vi "capex instrument control.vi"(0 "Keithley2268Lib.IKeithley2268":refnum<k7>, 4 "VISA resource name":refnum<visa-resource-name>, 6 "Bool in":bool[](array[boolean]), 7 "error in":errorcluster, 8 "Value in":dbl[](array[numeric]), 9 "Module":dbl=5.0, 10 "read/write":enum16{"read", "write"}(ring), 11 "Subsystem":T1(ring)=enum."temperature") -> (2 "Bool out":bool[](array[boolean]), 3 "Value out":dbl[](array[numeric]), 5 "error out":errorcluster)   [LabVIEW 2013]
uses:
  <vilib>/DAQmx/read.llb/DAQmx Read (Digital 1D Bool NChan 1Samp 1Line).vi
  <vilib>/DAQmx/write.llb/DAQmx Write (Digital 1D Bool NChan 1Samp 1Line).vi
  <vilib>/DAQmx/read.llb/DAQmx Read (Analog 2D DBL NChan NSamp).vi
  <vilib>/DAQmx/read.llb/DAQmx Read (Analog 1D DBL NChan 1Samp).vi
  <vilib>/DAQmx/write.llb/DAQmx Write (Analog 1D DBL NChan 1Samp).vi
  <vilib>/DAQmx/create/channels.llb/DAQmx Create Channel (DI-Digital Input).vi
  <vilib>/DAQmx/miscellaneous.llb/DAQmx Fill In Error Info.vi
  <vilib>/DAQmx/create/channels.llb/DAQmx Create Channel (DO-Digital Output).vi
  <vilib>/DAQmx/create/channels.llb/DAQmx Create Channel (AI-Temperature-Thermocouple).vi
  <vilib>/DAQmx/configure/timing.llb/DAQmx Timing (Sample Clock).vi
  <vilib>/DAQmx/create/channels.llb/DAQmx Create Channel (AI-Voltage-Basic).vi
  <vilib>/DAQmx/create/channels.llb/DAQmx Create Channel (AO-Voltage-Basic).vi
  <resource>/objmgr/daqmx.rc
  <instrlib>/APS-7000 Series/APS-7000 Series.lvlib
panel:
  in  "TC milliseconds to wait":u32=500
  out "Numeric 2":i32=12
  out "Numeric":i32=6
  in  "stop 5":bool
  in  "stop":bool
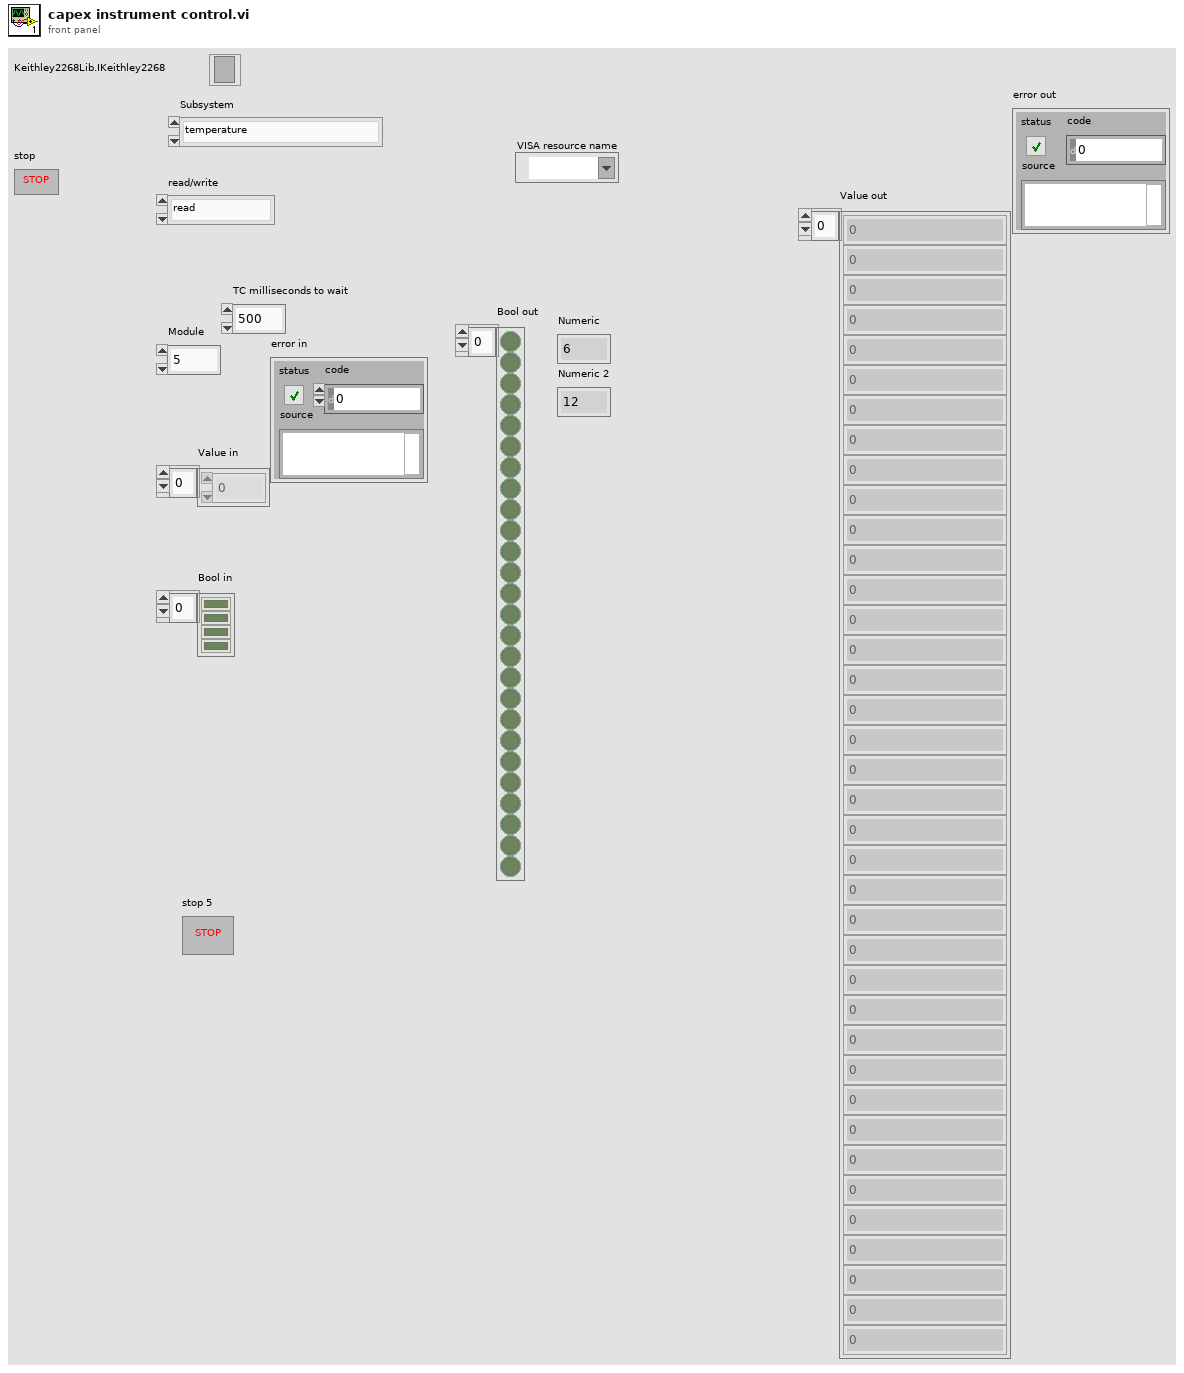
[diagram p1: front panel]
types:
  T1 = enum16{"Chiller", "Chamber", "DC power", "AC power", "GPIO", "temperature", "relays", "analog"}
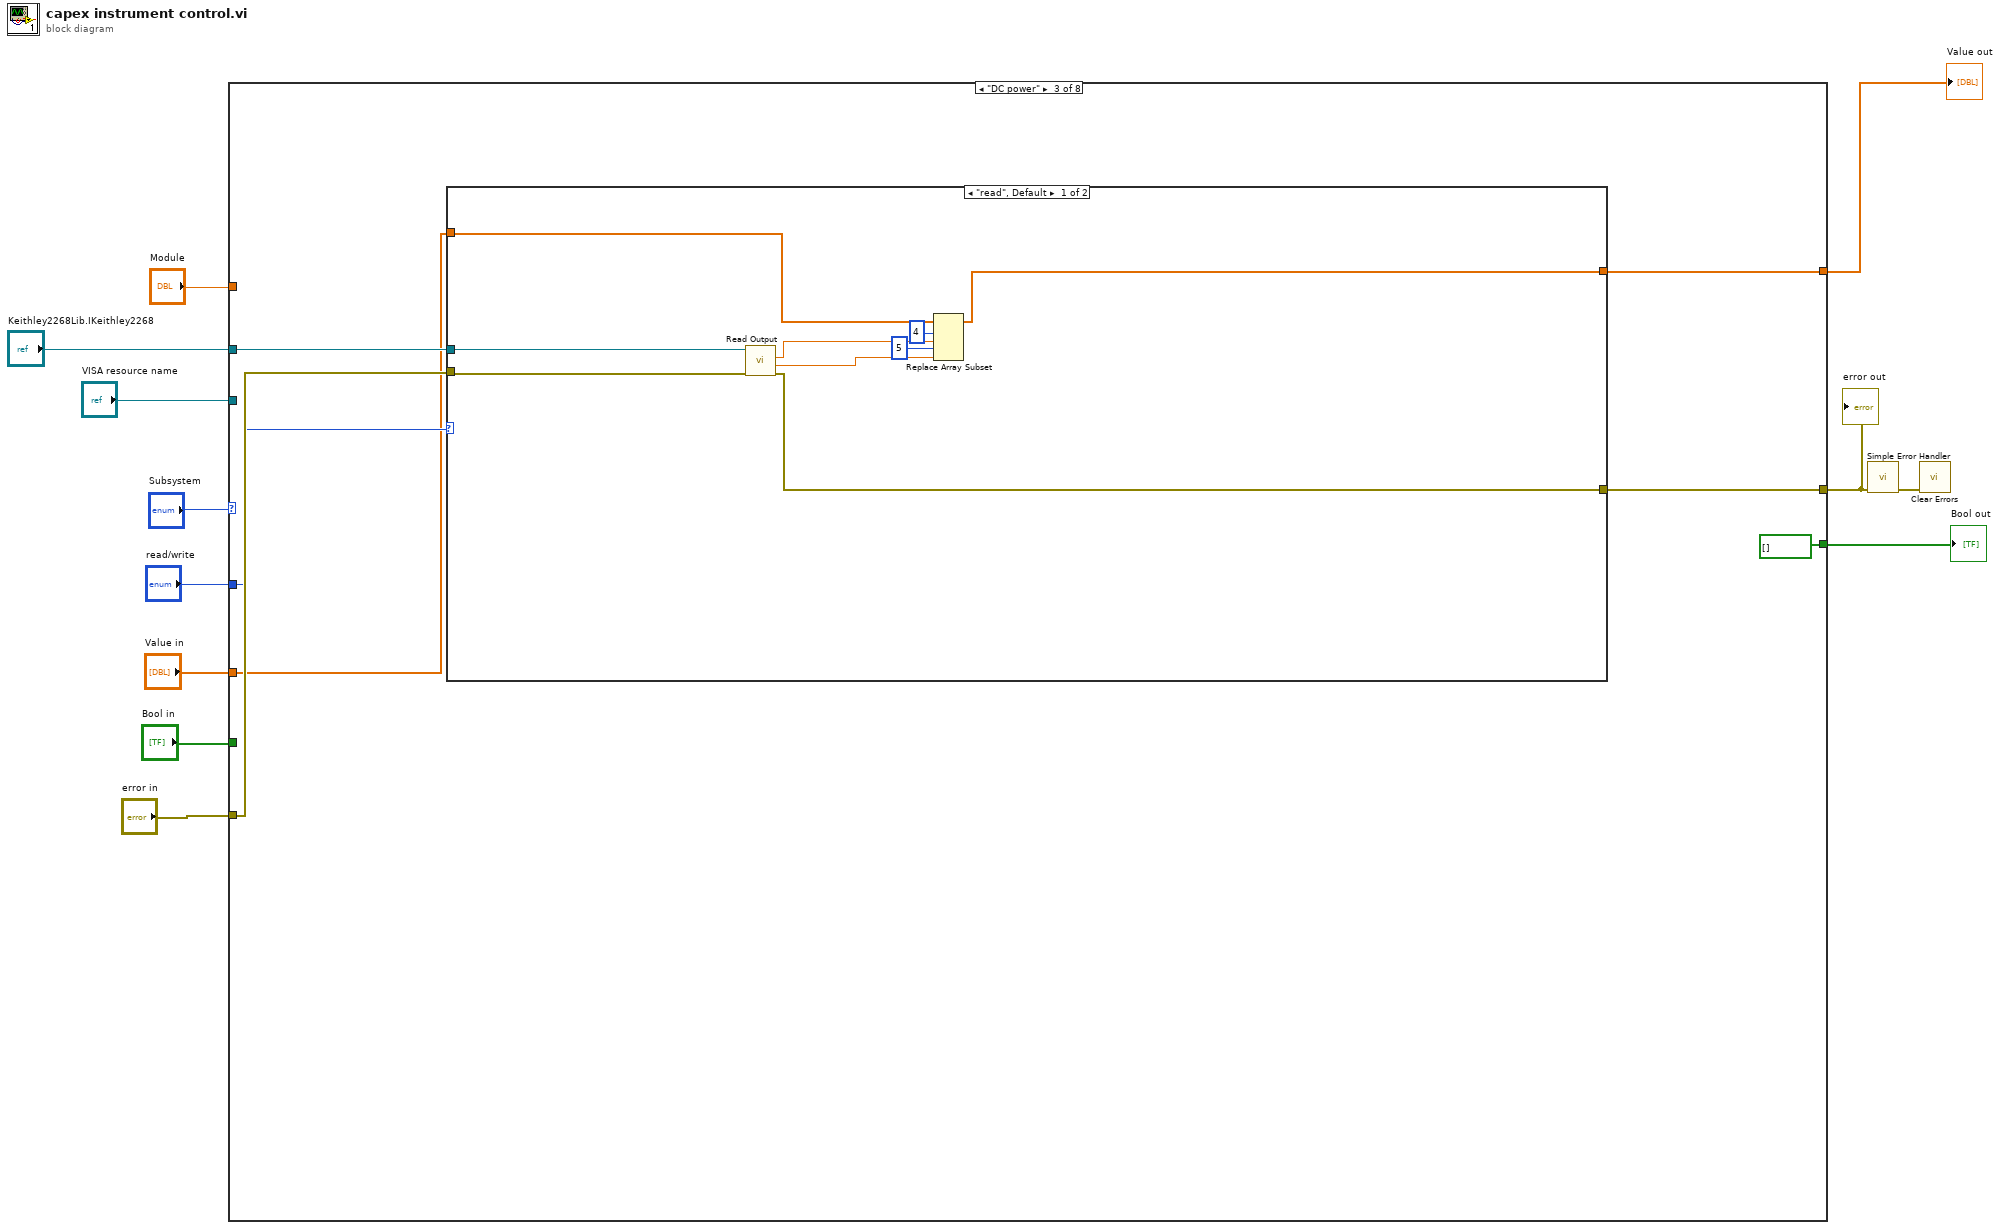
[diagram p0: block diagram]
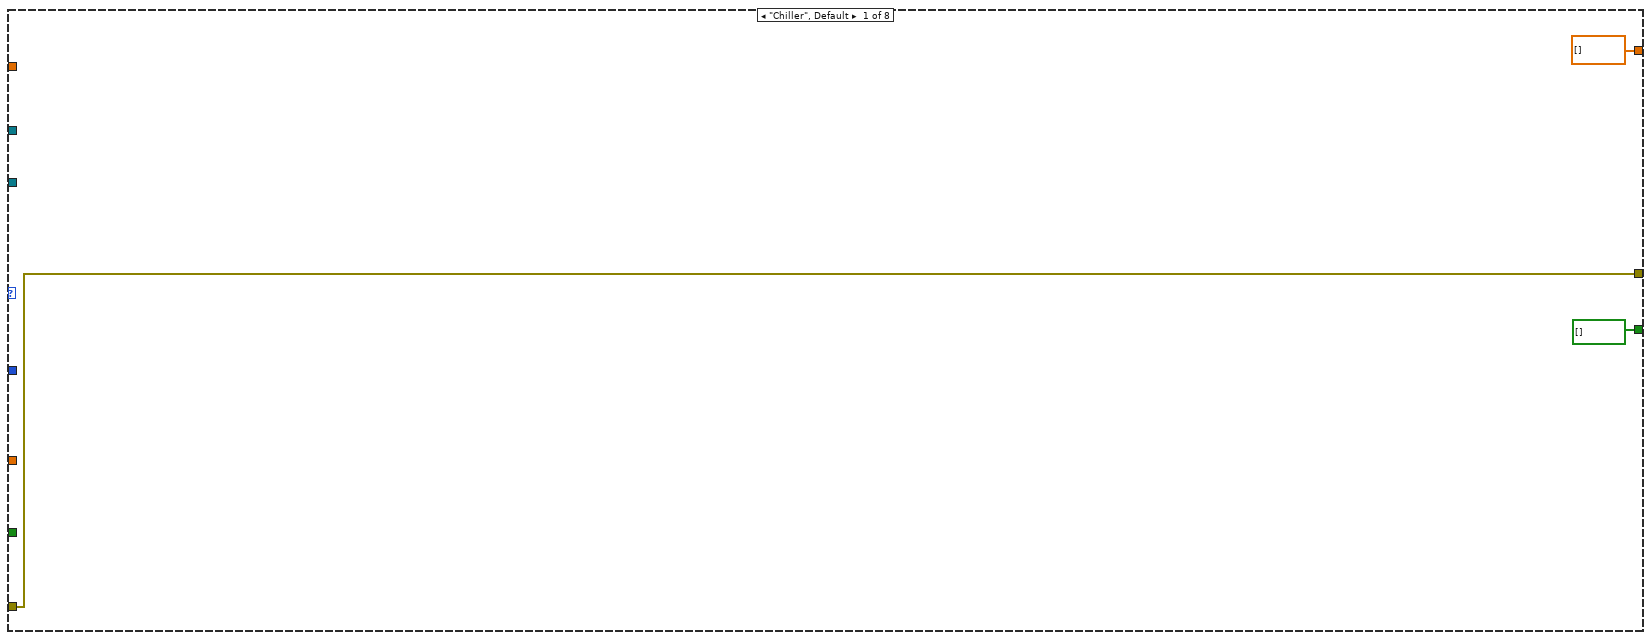
[diagram p2: hidden frame]
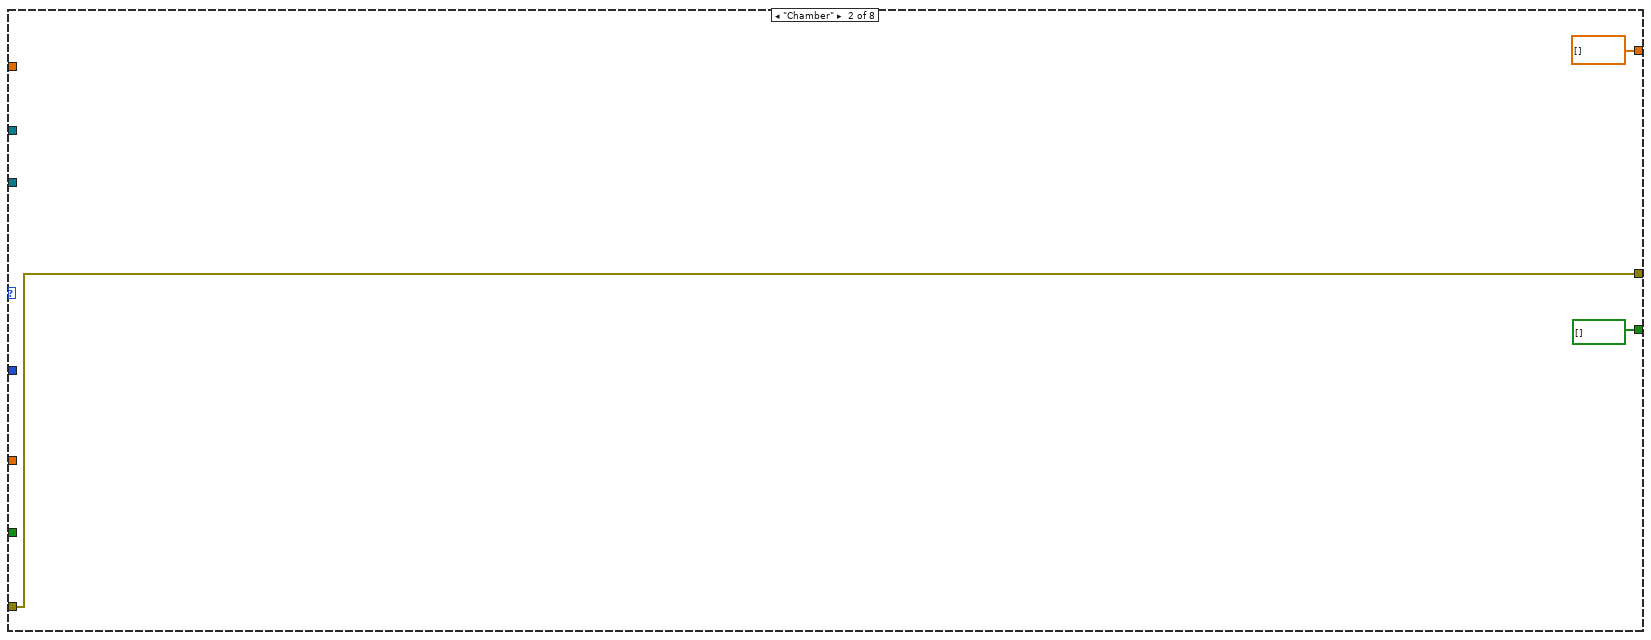
[diagram p3: hidden frame]
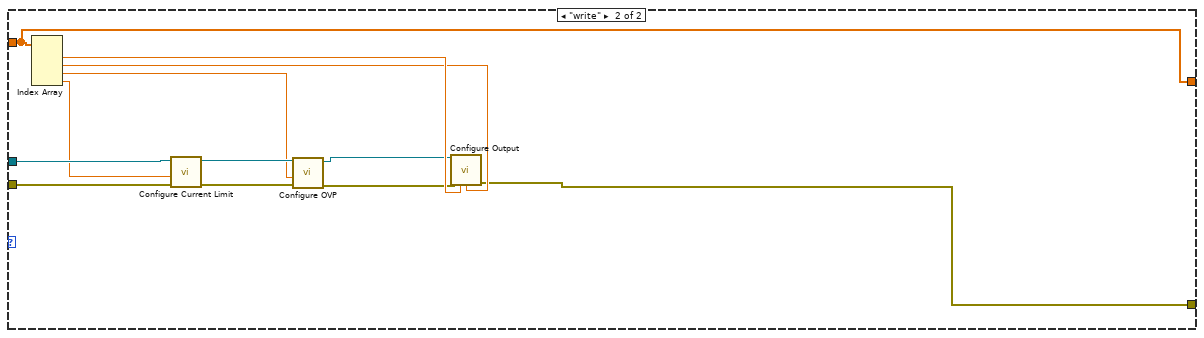
[diagram p4: hidden frame]
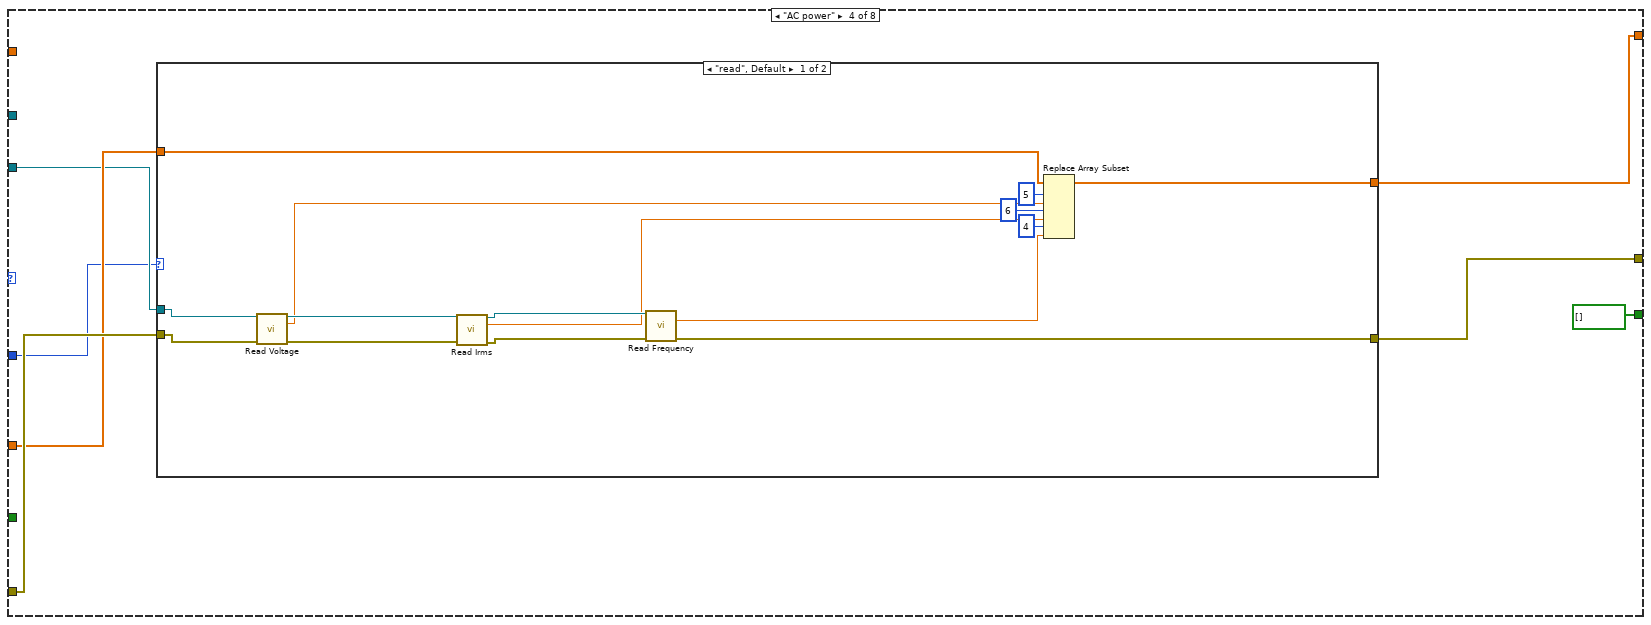
[diagram p5: hidden frame]
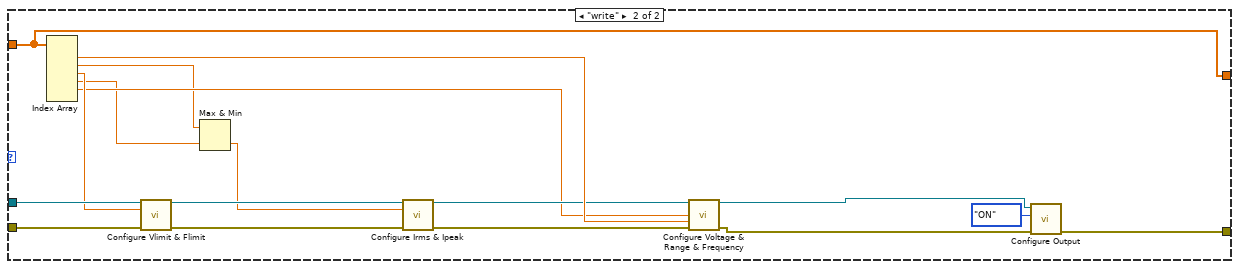
[diagram p6: hidden frame]
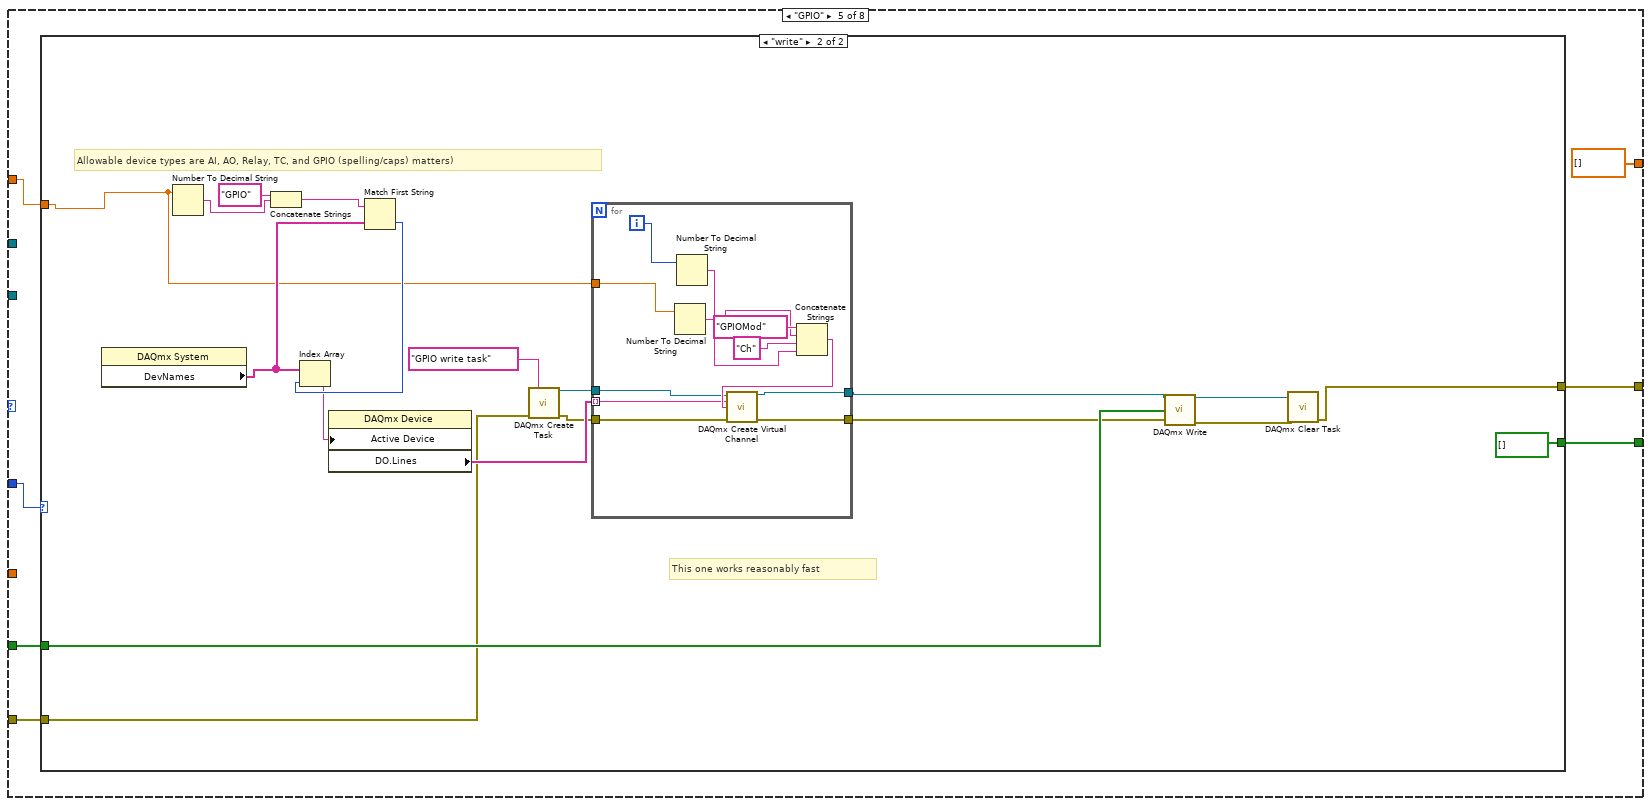
[diagram p7: hidden frame]
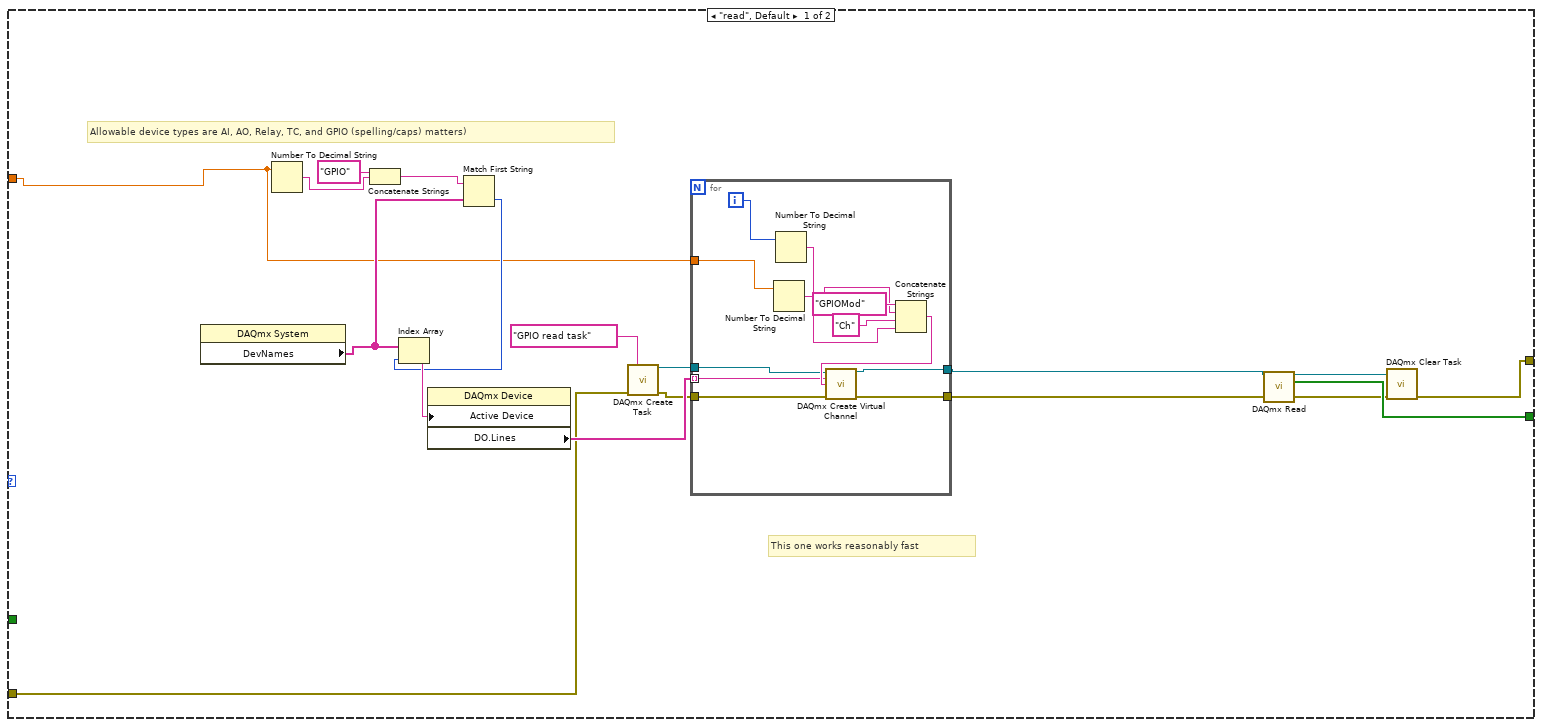
[diagram p8: hidden frame]
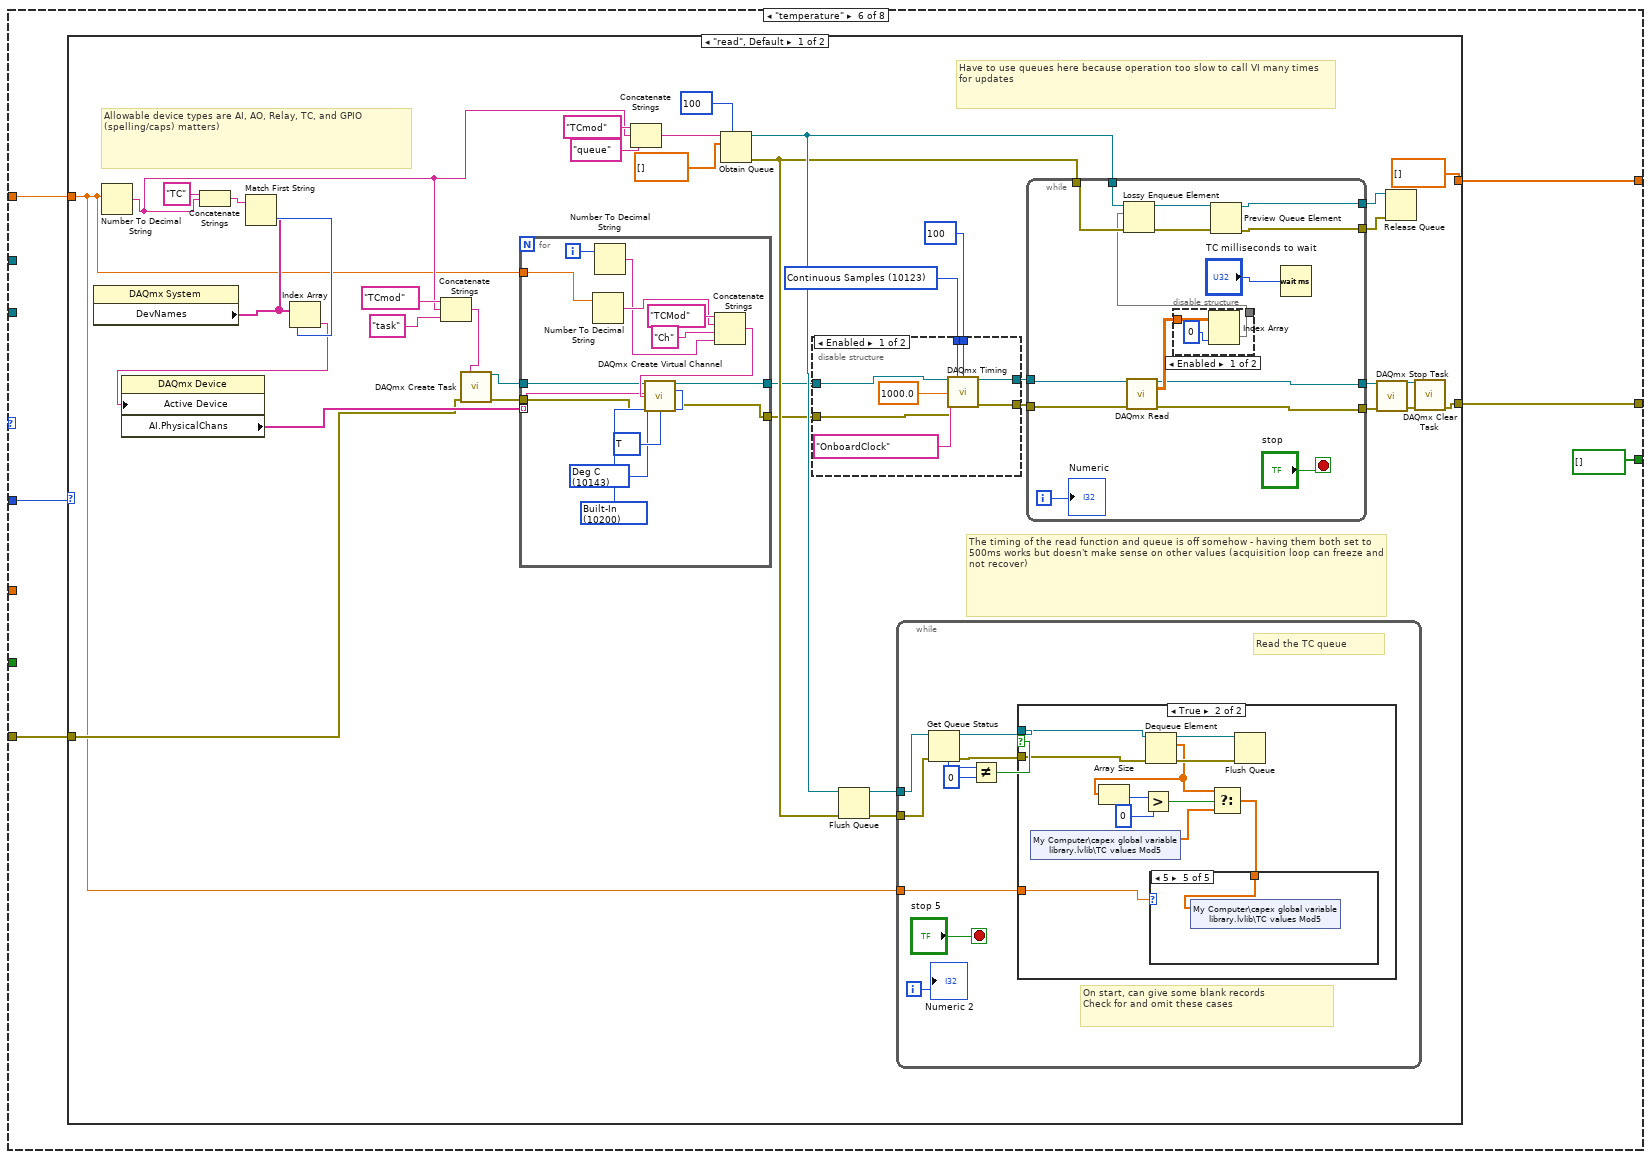
[diagram p9: hidden frame]
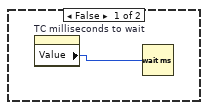
[diagram p11: hidden frame]
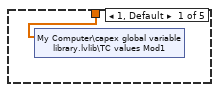
[diagram p12: hidden frame]
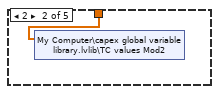
[diagram p13: hidden frame]
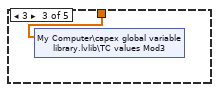
[diagram p14: hidden frame]
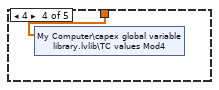
[diagram p15: hidden frame]
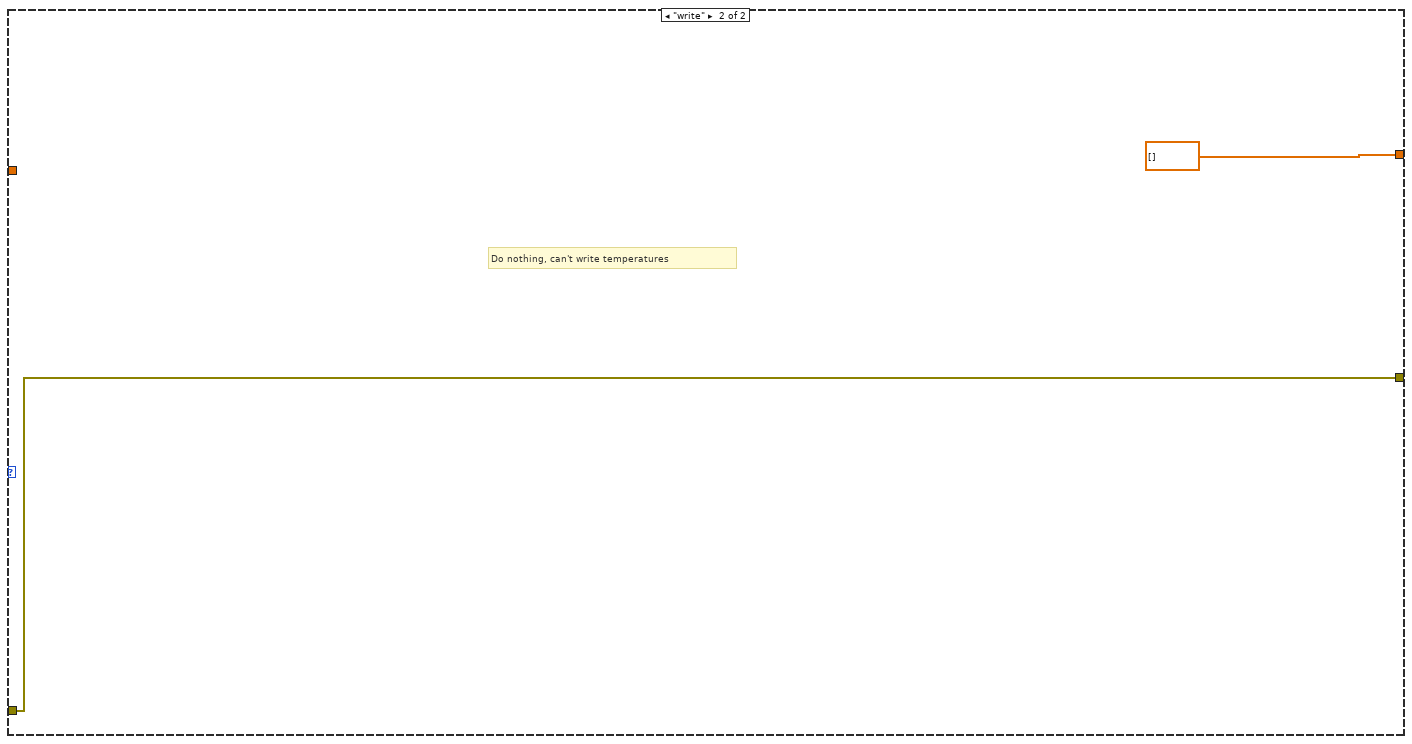
[diagram p17: hidden frame]
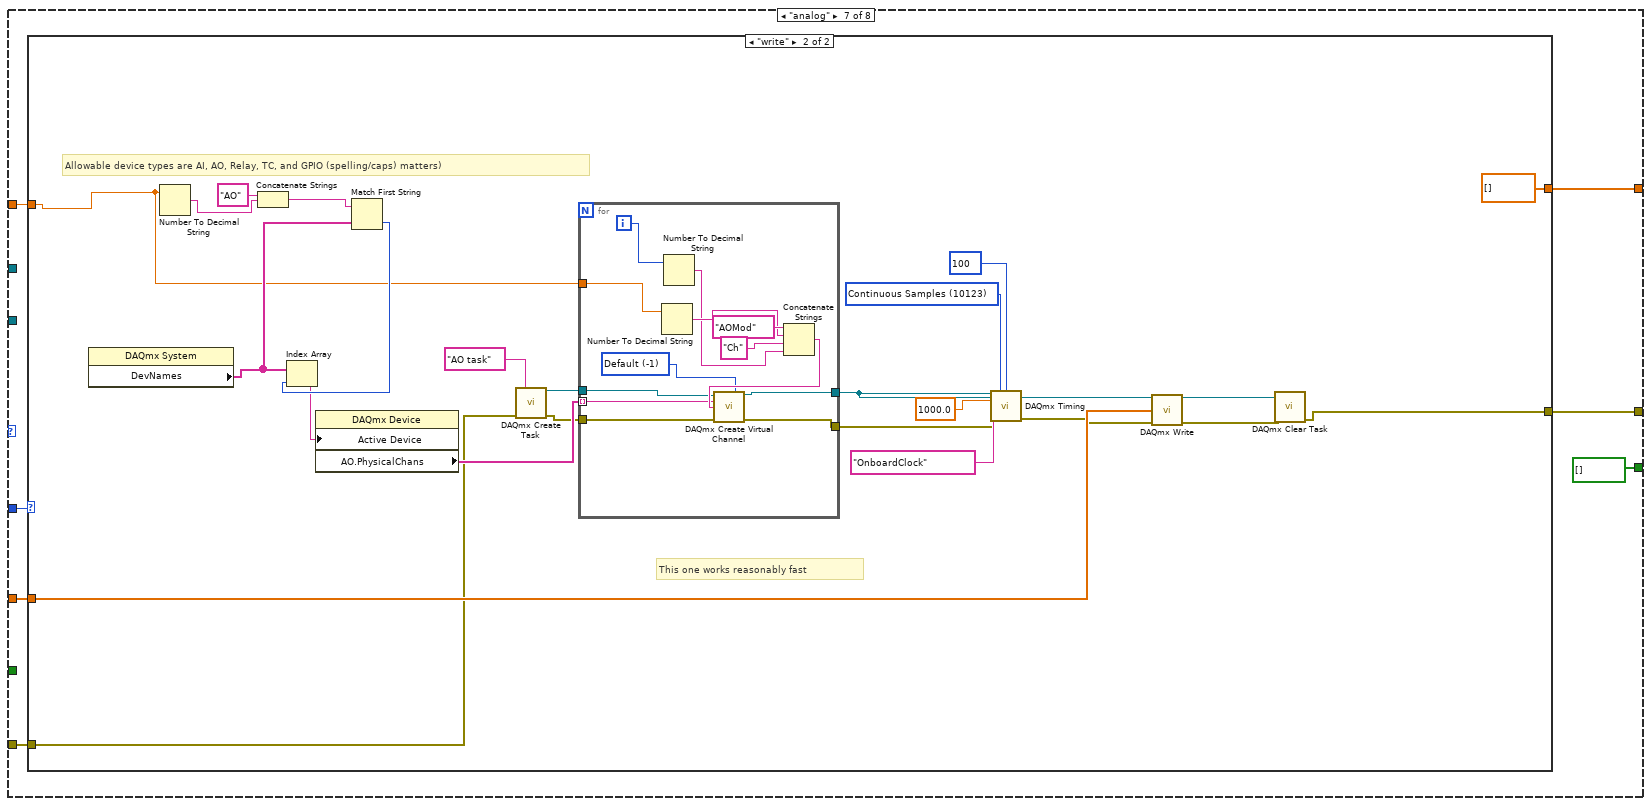
[diagram p18: hidden frame]
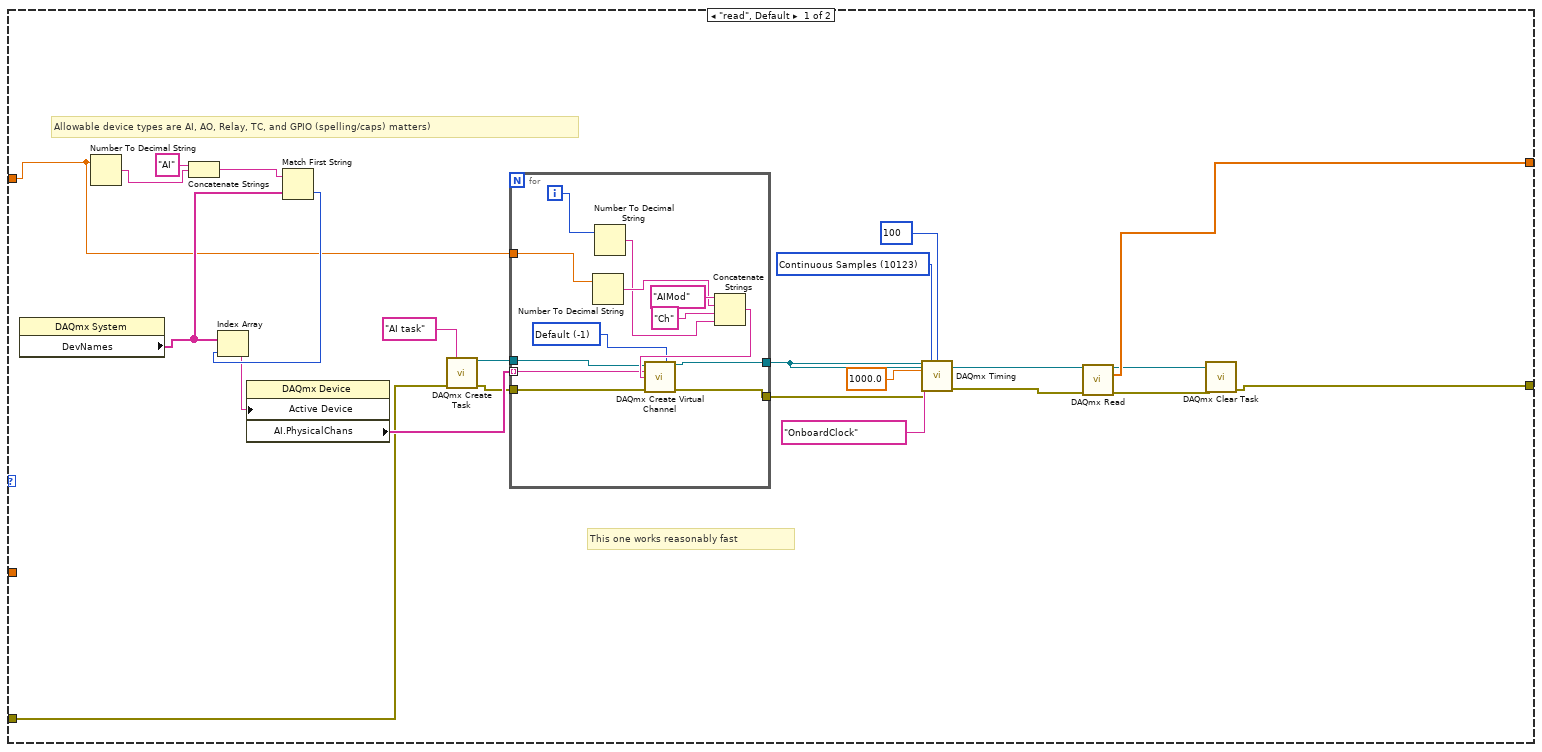
[diagram p19: hidden frame]
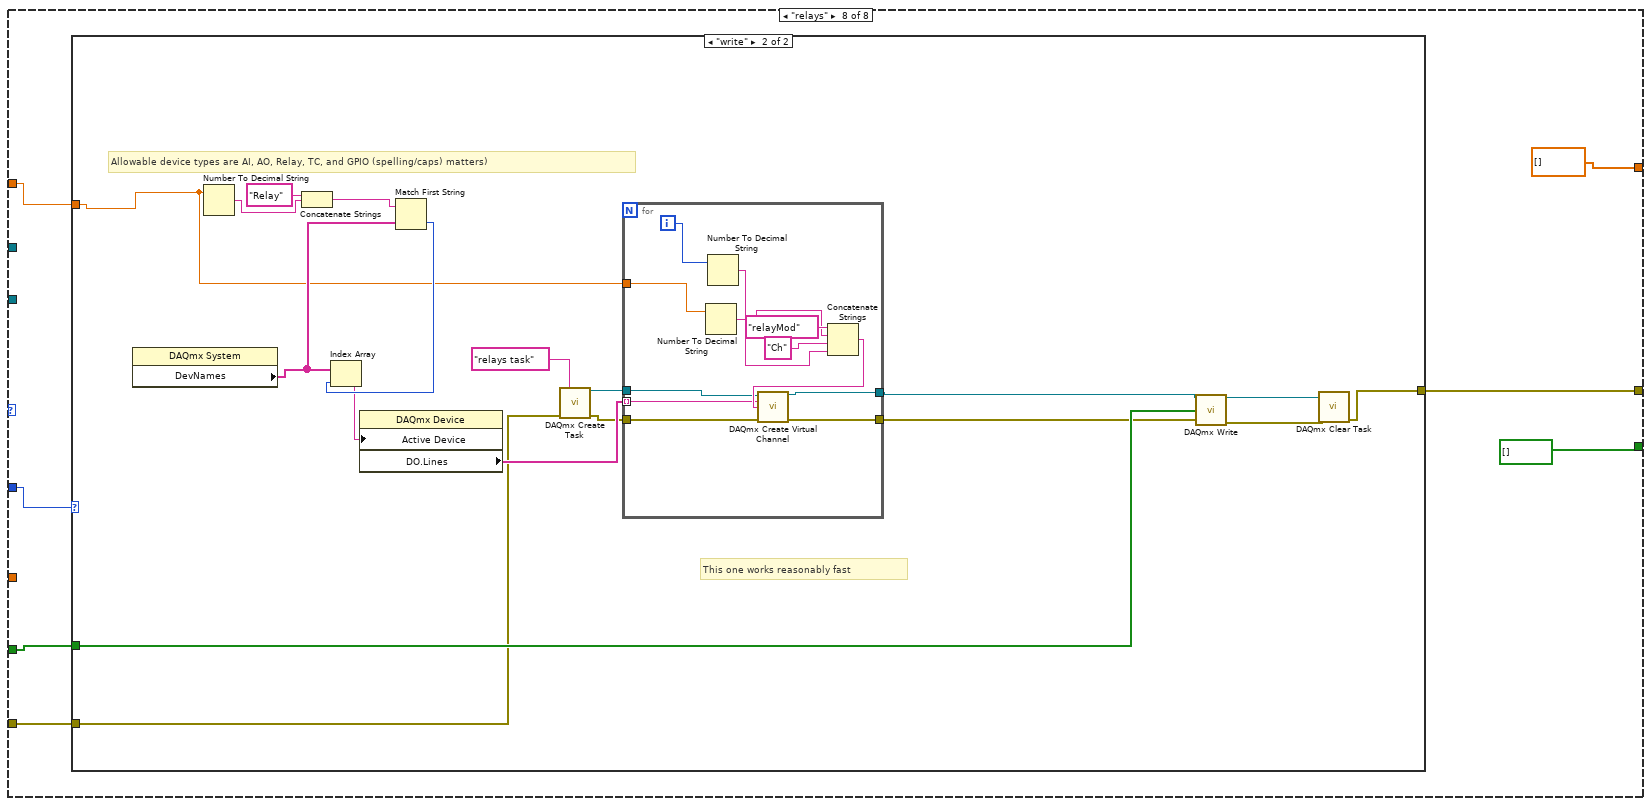
[diagram p20: hidden frame]
diagram:
  n1 = case shown="\"DC power\"" "Subsystem" {
    tunnel: "read/write" -> [_ _ w21 w48 w88 w159 w276 w352]
    tunnel: "Module" -> [_ _ _ _ w91 w158 w274 w356]
    tunnel: [dbl[] [] dbl[] [] w20 w47 dbl[] [] w157 w275 dbl[] []] -> w9
    tunnel: "Value in" -> [_ _ w19 w50 _ _ w273 _]
    tunnel: "Bool in" -> [_ _ _ _ w90 _ _ w355]
    tunnel: [bool[] [] ("data") bool[] [] ("data") bool[] [] ("data") bool[] [] ("data") w89 bool[] [] ("data") bool[] [] ("data") bool[] [] ("data")] -> w6
    tunnel: "error in" -> [w13 w16 w23 w52 w87 w155 w271 w351]
    tunnel: [w13 w16 w22 w51 w86 w154 w270 w350] -> w4
    tunnel: "VISA resource name" -> [_ _ _ w49 _ _ _ _]
    tunnel: "Keithley2268Lib.IKeithley2268" -> [_ _ w24 _ _ _ _ _]
    frame "Chiller", Default {
    }
    frame "Chamber" {
    }
    frame "DC power" {
      n2 = case shown="\"read\", Default" w21 {
        tunnel: w19 -> [w32 w35]
        tunnel: w24 -> [w34 w46]
        tunnel: w23 -> [w33 w39]
        tunnel: [w26 w36] -> w22
        tunnel: [w27 w35] -> w20
        frame "read", Default {
          n3 = call <instrlib>:"Read Output.vi"("error in (no error)"=w33, "Keithley2268Lib.IKeithley2268"=w34) -> ("error out"=w26:errorcluster, "Current Level (A)"=w29:dbl, "Voltage Level (V)"=w31:dbl)  [unwired: 6 in, 1 out]
          n4 = Replace Array Subset(array=w32, new element #1=w31, index #1=4 ("index"), new element #2=w29, index #2=5 ("index")) -> (w27:dbl[])
        }
        frame "write" {
          n5 = Index Array(array=w35) -> (element #1=w45:dbl, element #2=w44:dbl, element #3=w40:dbl, element #4=w41:dbl)  [unwired: 4 in]
          n6 = call <instrlib>:"Configure Current Limit.vi"("error in (no error)"=w39, "Current Limit (V)"=w41, "Keithley2268Lib.IKeithley2268"=w46) -> ("error out"=w38:errorcluster, "Keithley2268Lib.IKeithley2268"=w43:refnum<k7>)  [unwired: 7 in]
          n7 = call <instrlib>:"Configure OVP.vi"("error in (no error)"=w38, "OVP Level (V)"=w40, "Keithley2268Lib.IKeithley2268"=w43) -> ("error out"=w37:errorcluster, "Keithley2268Lib.IKeithley2268"=w42:refnum<k7>)  [unwired: 7 in]
          n8 = call <instrlib>:"Configure Output.vi"("Keithley2268Lib.IKeithley2268"=w42, "error in (no error)"=w37, "Voltage Level (V)"=w45, "Current Level (A)"=w44) -> ("error out"=w36:errorcluster)  [unwired: 10 in, 1 out]
        }
      }
    }
    frame "AC power" {
      n9 = case shown="\"read\", Default" w48 {
        tunnel: w52 -> [w64 w85]
        tunnel: [w61 w81] -> w51
        tunnel: w50 -> [w68 w69]
        tunnel: w49 -> [w67 w78]
        tunnel: [w54 w69] -> w47
        frame "read", Default {
          n10 = call <instrlib>:"Read Voltage.vi"("VISA session"=w67, "error in"=w64) -> ("dup VISA session"=w66:refnum<visa-resource-name>, "ACV?"=w60:dbl, "error out"=w63:errorcluster)  [unwired: 9 in, 2 out]
          n11 = call <instrlib>:"Read Irms.vi"("VISA in"=w66, "error in"=w63) -> ("VISA out"=w65:refnum<visa-resource-name>, "Irms? (Arms)"=w59:dbl, "error out"=w62:errorcluster)  [unwired: 9 in, 2 out]
          n12 = call <instrlib>:"Read Frequency.vi"("VISA session"=w65, "error in"=w62) -> ("Freq? (Hz)"=w58:dbl, "error out"=w61:errorcluster)  [unwired: 9 in, 3 out]
          n13 = Replace Array Subset(array=w68, new element #1=w60, index #1=5 ("index"), new element #2=w59, index #2=6 ("index"), new element #3=w58, index #3=4 ("index")) -> (w54:dbl[])
        }
        frame "write" {
          n14 = Index Array(array=w69) -> (element #1=w79:dbl, element #2=w72:dbl, element #3=w74:dbl, element #4=w71:dbl, element #5=w73:dbl)  [unwired: 6 in, 1 out]
          n15 = call <instrlib>:"Configure Vlimit & Flimit.vi"("VISA in"=w78, "Vlimit (Vrms)"=w74, "error in"=w85) -> ("VISA out"=w77:refnum<visa-resource-name>, "error out"=w84:errorcluster)  [unwired: 5 in, 6 out]
          n16 = Max & Min(x=w72, y=w71) -> (min(x,y)=w70:dbl)  [unwired: 1 out]
          n17 = call <instrlib>:"Configure Irms & Ipeak.vi"("VISA in"=w77, "Irms (A)"=w70, "error in"=w84) -> ("VISA out"=w76:refnum<visa-resource-name>, "error out"=w83:errorcluster)  [unwired: 5 in, 6 out]
          n18 = call <instrlib>:"Configure Voltage & Range & Frequency.vi"("VISA in"=w76, "FREQ"=w73, "ACV"=w79, "error in"=w83) -> ("VISA out"=w75:refnum<visa-resource-name>, "error out"=w82:errorcluster)  [unwired: 3 in, 7 out]
          n19 = call <instrlib>:"Configure Output.vi"("error in"=w82, "Output ON/OFF"=enum16{"OFF", "ON"}."ON", "VISA in"=w75) -> ("error out"=w81:errorcluster)  [unwired: 6 in, 2 out]
        }
      }
    }
    frame "GPIO" {
      n20 = case shown="\"write\"" w88 {
        tunnel: w91 -> [w100 w131]
        tunnel: w90 -> [_ w130]
        tunnel: [w99 bool[] [] ("data")] -> w89
        tunnel: w87 -> [w97 w127]
        tunnel: [w93 w123] -> w86
        frame "read", Default {
          # "Allowable device types are AI, AO, Relay, TC, and GPIO (spelling/caps) matters)"
          # "This one works reasonably fast"
          n21 = property class="DAQmx System"() -> ("DevNames"=w105:tag[])  [unwired: 2 in, 2 out]
          n22 = Number To Decimal String(number=w100) -> (decimal integer string=w102:string)  [unwired: 1 in]
          n23 = Concatenate Strings("GPIO" ("string"), w102) -> (w103:string)
          n24 = Match First String(2:w105, 3:w103) -> (0:w104:i32)  [unwired: 1 out]
          n25 = Index Array(array=w105, index=w104) -> (element=w106:tag)
          n26 = property class="DAQmx Device"("Active Device"=w106) -> ("DO.Lines"=w109:tag[])  [unwired: 2 in, 2 out]
          n27 = call <vilib>:"DAQmx Create Task.vi"("new task name"="GPIO read task", "error in"=w97) -> ("task out"=w107:refnum<k21>, "error out"=w96:errorcluster)  [unwired: 12 in]
          n28 = for {
            tunnel: w100 -> [w117]
            tunnel: w107 -> [w116]
            tunnel: [w115] -> w98
            tunnel: w109 -> [w114] mode=indexing
            tunnel: w96 -> [w112]
            tunnel: [w111] -> w95
            i -> [w113]
            n29 = Number To Decimal String(number=w117) -> (decimal integer string=w121:string)  [unwired: 1 in]
            n30 = Number To Decimal String(number=w113) -> (decimal integer string=w120:string)  [unwired: 1 in]
            n31 = Concatenate Strings("GPIOMod" ("string"), w121, "Ch" ("string"), w120) -> (w118:string)
            n32 = call-poly <vilib>:"DAQmx Create Virtual Channel.vi"("task in"=w116, "lines"=w114, "name to assign"=w118, "error in"=w112) -> ("task out"=w115:refnum<k21>, "error out"=w111:errorcluster)  [unwired: 10 in]
          }
          n33 = call-poly <vilib>:"DAQmx Read.vi"("task/channels in"=w98, "error in"=w95) -> ("task out"=w108:refnum<k21>, "data"=w99:bool[], "error out"=w94:errorcluster)  [unwired: 11 in]
          n34 = call <vilib>:"DAQmx Clear Task.vi"("task in"=w108, "error in"=w94) -> ("error out"=w93:errorcluster)  [unwired: 13 in]
        }
        frame "write" {
          # "Allowable device types are AI, AO, Relay, TC, and GPIO (spelling/caps) matters)"
          # "This one works reasonably fast"
          n35 = property class="DAQmx System"() -> ("DevNames"=w137:tag[])  [unwired: 2 in, 2 out]
          n36 = Number To Decimal String(number=w131) -> (decimal integer string=w140:string)  [unwired: 1 in]
          n37 = Concatenate Strings("GPIO" ("string"), w140) -> (w139:string)
          n38 = Match First String(2:w137, 3:w139) -> (0:w138:i32)  [unwired: 1 out]
          n39 = Index Array(array=w137, index=w138) -> (element=w136:tag)
          n40 = property class="DAQmx Device"("Active Device"=w136) -> ("DO.Lines"=w133:tag[])  [unwired: 2 in, 2 out]
          n41 = call <vilib>:"DAQmx Create Task.vi"("new task name"="GPIO write task", "error in"=w127) -> ("task out"=w135:refnum<k21>, "error out"=w126:errorcluster)  [unwired: 12 in]
          n42 = for {
            tunnel: w131 -> [w148]
            tunnel: w135 -> [w147]
            tunnel: [w146] -> w128
            tunnel: w133 -> [w145] mode=indexing
            tunnel: w126 -> [w143]
            tunnel: [w142] -> w125
            i -> [w144]
            n43 = Number To Decimal String(number=w148) -> (decimal integer string=w152:string)  [unwired: 1 in]
            n44 = Number To Decimal String(number=w144) -> (decimal integer string=w151:string)  [unwired: 1 in]
            n45 = Concatenate Strings("GPIOMod" ("string"), w152, "Ch" ("string"), w151) -> (w149:string)
            n46 = call-poly <vilib>:"DAQmx Create Virtual Channel.vi"("task in"=w147, "lines"=w145, "name to assign"=w149, "error in"=w143) -> ("task out"=w146:refnum<k21>, "error out"=w142:errorcluster)  [unwired: 10 in]
          }
          n47 = call-poly <vilib>:"DAQmx Write.vi"("task/channels in"=w128, "data"=w130, "error in"=w125) -> ("task out"=w134:refnum<k21>, "error out"=w124:errorcluster)  [unwired: 10 in, 1 out]
          n48 = call <vilib>:"DAQmx Clear Task.vi"("task in"=w134, "error in"=w124) -> ("error out"=w123:errorcluster)  [unwired: 13 in]
        }
      }
    }
    frame "temperature" {
      n49 = case shown="\"read\", Default" w159 {
        tunnel: w158 -> [w174 _]
        tunnel: [dbl[] [] dbl[] []] -> w157
        tunnel: w155 -> [w190 w268]
        tunnel: [w169 w268] -> w154
        frame "read", Default {
          w168 = 10123 items=["Finite Samples"=10178, "Continuous Samples"=10123, "Hardware Timed Single Point"=12522] ("sample mode")
          # "The timing of the read function and queue is off somehow - having them both set to 500ms works but doesn't make sense on other values (acquisition loop can freeze and not recover)"
          # "Have to use queues here because operation too slow to call VI many times for updates"
          # "Allowable device types are AI, AO, Relay, TC, and GPIO (spelling/caps) matters)"
          n50 = property class="DAQmx System"() -> ("DevNames"=w194:tag[])  [unwired: 2 in, 2 out]
          n51 = Number To Decimal String(number=w174) -> (decimal integer string=w181:string)  [unwired: 1 in]
          n52 = Concatenate Strings("TC" ("string"), w181) -> (w178:string)
          n53 = Match First String(2:w194, 3:w178) -> (0:w195:i32)  [unwired: 1 out]
          n54 = Index Array(array=w194, index=w195) -> (element=w193:tag)
          n55 = property class="DAQmx Device"("Active Device"=w193) -> ("AI.PhysicalChans"=w191:tag[])  [unwired: 2 in, 2 out]
          n56 = Concatenate Strings("TCmod" ("new task name"), w181, "task" ("string")) -> (w179:string)
          n57 = call <vilib>:"DAQmx Create Task.vi"("new task name"=w179, "error in"=w190) -> ("task out"=w192:refnum<k21>, "error out"=w189:errorcluster)  [unwired: 12 in]
          n58 = for {
            tunnel: w174 -> [w267]
            tunnel: [w258] -> w165
            tunnel: w192 -> [w256]
            tunnel: w191 -> [w255] mode=indexing
            tunnel: w189 -> [w254]
            tunnel: [w253] -> w166
            i -> [w257]
            w259 = 10200 items=["Built-In"=10200, "Constant Value"=10116, "Channel"=10113] ("cjc source")
            w260 = 10143 items=["Deg C"=10143, "Deg F"=10144, "Kelvins"=10325, "Deg R"=10145, "From Custom Scale"=10065] ("units")
            w266 = 10086 items=["J"=10072, "K"=10073, "N"=10077, "R"=10082, "S"=10085, "T"=10086, "B"=10047, "E"=10055] ("thermocouple type")
            n59 = Number To Decimal String(number=w267) -> (decimal integer string=w264:string)  [unwired: 1 in]
            n60 = Number To Decimal String(number=w257) -> (decimal integer string=w263:string)  [unwired: 1 in]
            n61 = Concatenate Strings("TCMod" ("string"), w264, "Ch" ("string"), w263) -> (w261:string)
            n62 = call-poly <vilib>:"DAQmx Create Virtual Channel.vi"("task in"=w256, "physical channels"=w255, "cjc source"=w259, "name to assign"=w261, "units"=w260, "error in"=w254, "thermocouple type"=w266) -> ("task out"=w258:refnum<k21>, "error out"=w253:errorcluster)  [unwired: 7 in]
          }
          n63 = Concatenate Strings("TCmod" ("string"), w181, "queue" ("string")) -> (w186:string)
          n64 = Obtain Queue(max queue size (-1, unlimited)=100, name (unnamed)=w186, element data type=dbl[] [] ("Value out 2")) -> (queue out=w176:refnum<queue>, error out=w175:errorcluster)  [unwired: 2 in, 1 out]
          n65 = disable-structure shown="Enabled" {
            disable-tunnel: w168 -> [w202 _]
            disable-tunnel: 100 ("samples per channel") -> [w201 _]
            disable-tunnel: w166 -> [w200 w205]
            disable-tunnel: w165 -> [w199 w206]
            disable-tunnel: [w198 w206] -> w164
            disable-tunnel: [w197 w205] -> w163
            frame Enabled {
              n66 = call-poly <vilib>:"DAQmx Timing.vi"("task/channels in"=w199, "sample mode"=w202, "samples per channel"=w201, "rate"=1000.0, "source"=tag "OnboardClock", "error in"=w200) -> ("task out"=w198:refnum<k21>, "error out"=w197:errorcluster)  [unwired: 8 in]
            }
            frame Disabled {
            }
          }
          n67 = Flush Queue(queue=w176, error in (no error)=w175) -> (queue out=w161:refnum<queue>, error out=w160:errorcluster)  [unwired: 1 out]
          n68 = while {
            tunnel: w161 -> [w213]
            tunnel: w160 -> [w212]
            tunnel: w174 -> [w208]
            i -> [w215]
            stop <- "stop 5" stop-if-true
            # "On start, can give some blank records\nCheck for and omit these cases"
            # "Read the TC queue"
            n69 = Get Queue Status(queue=w213, error in (no error)=w212) -> (queue out=w210:refnum<queue>, error out=w209:errorcluster, # elements in queue=w207:i32)  [unwired: 1 in, 5 out]
            n70 = Not Equal?(x=w207, y=0) -> (x != y?=w211:bool)
            n71 = case shown="True" w211 {
              tunnel: w210 -> [_ w226]
              tunnel: w209 -> [_ w225]
              tunnel: w208 -> [_ w224]
              frame False {
                n72 = property on="TC milliseconds to wait" class="DigNum (strict)"() -> ("Value"=w217:u32)  [unwired: 2 in, 2 out]
                n73 = Wait (ms)(milliseconds to wait=w217) -> ()  [unwired: 1 out]
              }
              frame True {
                n74 = shared-variable "My Computer\\capex global variable library.lvlib\\TC values Mod5"() -> (w218:dbl[])  [unwired: 1 in, 1 out]
                n75 = Dequeue Element(queue=w226, error in (no error)=w225) -> (queue out=w228:refnum<queue>, element=w220:dbl[], error out=w227:errorcluster)  [unwired: 1 in, 1 out]
                n76 = Array Size(array=w220) -> (size(s)=w223:i32)
                n77 = Greater?(x=w223, y=0) -> (0:w221:bool)
                n78 = Select(t=w220, s=w221, f=w218) -> (s? t:f=w219:dbl[])
                n79 = case shown="5" w224 {
                  tunnel: w219 -> [w229 w230 w231 w232 w233]
                  frame 1, Default {
                    n80 = shared-variable "My Computer\\capex global variable library.lvlib\\TC values Mod1"(w229) -> ()  [unwired: 1 in, 1 out]
                  }
                  frame 2 {
                    n81 = shared-variable "My Computer\\capex global variable library.lvlib\\TC values Mod2"(w230) -> ()  [unwired: 1 in, 1 out]
                  }
                  frame 3 {
                    n82 = shared-variable "My Computer\\capex global variable library.lvlib\\TC values Mod3"(w231) -> ()  [unwired: 1 in, 1 out]
                  }
                  frame 4 {
                    n83 = shared-variable "My Computer\\capex global variable library.lvlib\\TC values Mod4"(w232) -> ()  [unwired: 1 in, 1 out]
                  }
                  frame 5 {
                    n84 = shared-variable "My Computer\\capex global variable library.lvlib\\TC values Mod5"(w233) -> ()  [unwired: 1 in, 1 out]
                  }
                }
                n85 = Flush Queue(queue=w228, error in (no error)=w227) -> ()  [unwired: 3 out]
              }
            }
            "Numeric 2" <- w215
          }
          n86 = while {
            tunnel: [w236] -> w173
            tunnel: w163 -> [w240]
            tunnel: [w235] -> w172
            tunnel: w176 -> [w247]
            tunnel: [w245] -> w184
            tunnel: w175 -> [w246]
            tunnel: [w244] -> w183
            tunnel: w164 -> [w239]
            i -> [w241]
            stop <- "stop" stop-if-true
            n87 = call-poly <vilib>:"DAQmx Read.vi"("task/channels in"=w239, "error in"=w240) -> ("task out"=w236:refnum<k21>, "data"=w237:dbl[][], "error out"=w235:errorcluster)  [unwired: 11 in]
            n88 = disable-structure shown="Enabled" {
              disable-tunnel: [w251 w252] -> w238
              disable-tunnel: w237 -> [w249 w252]
              frame Enabled {
                n89 = Index Array(array=w249, index (col)=0 ("index (row)")) -> (element=w251:dbl[])  [unwired: 1 in]
              }
              frame Disabled {
              }
            }
            n90 = Lossy Enqueue Element(queue=w247, element=w238, error in (no error)=w246) -> (queue out=w243:refnum<queue>, error out=w242:errorcluster)  [unwired: 2 out]
            n91 = Preview Queue Element(queue=w243, error in (no error)=w242) -> (queue out=w245:refnum<queue>, error out=w244:errorcluster)  [unwired: 1 in, 2 out]
            n92 = Wait (ms)(milliseconds to wait="TC milliseconds to wait") -> ()  [unwired: 1 out]
            "Numeric" <- w241
          }
          n93 = call <vilib>:"DAQmx Stop Task.vi"("task/channels in"=w173, "error in"=w172) -> ("task out"=w171:refnum<k21>, "error out"=w170:errorcluster)  [unwired: 12 in]
          n94 = Release Queue(queue=w184, error in (no error)=w183) -> ()  [unwired: 1 in, 3 out]
          n95 = call <vilib>:"DAQmx Clear Task.vi"("task in"=w171, "error in"=w170) -> ("error out"=w169:errorcluster)  [unwired: 13 in]
        }
        frame "write" {
          # "Do nothing, can't write temperatures"
        }
      }
    }
    frame "analog" {
      n96 = case shown="\"write\"" w276 {
        tunnel: [w293 dbl[] []] -> w275
        tunnel: w274 -> [w292 w320]
        tunnel: w273 -> [_ w319]
        tunnel: w271 -> [w282 w318]
        tunnel: [w277 w313] -> w270
        frame "read", Default {
          w289 = 10123 items=["Finite Samples"=10178, "Continuous Samples"=10123, "Hardware Timed Single Point"=12522] ("sample mode")
          # "Allowable device types are AI, AO, Relay, TC, and GPIO (spelling/caps) matters)"
          # "This one works reasonably fast"
          n97 = property class="DAQmx System"() -> ("DevNames"=w295:tag[])  [unwired: 2 in, 2 out]
          n98 = Number To Decimal String(number=w292) -> (decimal integer string=w298:string)  [unwired: 1 in]
          n99 = Concatenate Strings("AI" ("string"), w298) -> (w297:string)
          n100 = Match First String(2:w295, 3:w297) -> (0:w296:i32)  [unwired: 1 out]
          n101 = Index Array(array=w295, index=w296) -> (element=w294:tag)
          n102 = property class="DAQmx Device"("Active Device"=w294) -> ("AI.PhysicalChans"=w284:tag[])  [unwired: 2 in, 2 out]
          n103 = call <vilib>:"DAQmx Create Task.vi"("new task name"="AI task", "error in"=w282) -> ("task out"=w291:refnum<k21>, "error out"=w281:errorcluster)  [unwired: 12 in]
          n104 = for {
            tunnel: w292 -> [w306]
            tunnel: w291 -> [w305]
            tunnel: [w304] -> w286
            tunnel: w284 -> [w303] mode=indexing
            tunnel: w281 -> [w301]
            tunnel: [w300] -> w280
            i -> [w302]
            w307 = -1 items=["Default"=-1, "RSE"=10083, "NRSE"=10078, "Differential"=10106, "Pseudodifferential"=12529] ("input terminal configuration")
            n105 = Number To Decimal String(number=w306) -> (decimal integer string=w311:string)  [unwired: 1 in]
            n106 = Number To Decimal String(number=w302) -> (decimal integer string=w310:string)  [unwired: 1 in]
            n107 = Concatenate Strings("AIMod" ("string"), w311, "Ch" ("string"), w310) -> (w308:string)
            n108 = call-poly <vilib>:"DAQmx Create Virtual Channel.vi"("task in"=w305, "input terminal configuration"=w307, "physical channels"=w303, "name to assign"=w308, "error in"=w301) -> ("task out"=w304:refnum<k21>, "error out"=w300:errorcluster)  [unwired: 9 in]
          }
          n109 = call-poly <vilib>:"DAQmx Timing.vi"("task/channels in"=w286, "sample mode"=w289, "samples per channel"=100, "rate"=1000.0, "source"=tag "OnboardClock", "error in"=w280) -> ("error out"=w279:errorcluster)  [unwired: 8 in, 1 out]
          n110 = call-poly <vilib>:"DAQmx Read.vi"("task/channels in"=w286, "error in"=w279) -> ("task out"=w285:refnum<k21>, "data"=w293:dbl[], "error out"=w278:errorcluster)  [unwired: 11 in]
          n111 = call <vilib>:"DAQmx Clear Task.vi"("task in"=w285, "error in"=w278) -> ("error out"=w277:errorcluster)  [unwired: 13 in]
        }
        frame "write" {
          w327 = 10123 items=["Finite Samples"=10178, "Continuous Samples"=10123, "Hardware Timed Single Point"=12522] ("sample mode")
          # "Allowable device types are AI, AO, Relay, TC, and GPIO (spelling/caps) matters)"
          # "This one works reasonably fast"
          n112 = property class="DAQmx System"() -> ("DevNames"=w331:tag[])  [unwired: 2 in, 2 out]
          n113 = Number To Decimal String(number=w320) -> (decimal integer string=w334:string)  [unwired: 1 in]
          n114 = Concatenate Strings("AO" ("string"), w334) -> (w333:string)
          n115 = Match First String(2:w331, 3:w333) -> (0:w332:i32)  [unwired: 1 out]
          n116 = Index Array(array=w331, index=w332) -> (element=w330:tag)
          n117 = property class="DAQmx Device"("Active Device"=w330) -> ("AO.PhysicalChans"=w322:tag[])  [unwired: 2 in, 2 out]
          n118 = call <vilib>:"DAQmx Create Task.vi"("new task name"="AO task", "error in"=w318) -> ("task out"=w329:refnum<k21>, "error out"=w317:errorcluster)  [unwired: 12 in]
          n119 = for {
            tunnel: w320 -> [w343]
            tunnel: w329 -> [w342]
            tunnel: [w341] -> w324
            tunnel: w322 -> [w340] mode=indexing
            tunnel: w317 -> [w338]
            tunnel: [w337] -> w316
            i -> [w339]
            w344 = -1 items=["Default"=-1, "RSE"=10083, "NRSE"=10078, "Differential"=10106, "Pseudodifferential"=12529] ("input terminal configuration")
            n120 = Number To Decimal String(number=w343) -> (decimal integer string=w348:string)  [unwired: 1 in]
            n121 = Number To Decimal String(number=w339) -> (decimal integer string=w347:string)  [unwired: 1 in]
            n122 = Concatenate Strings("AOMod" ("string"), w348, "Ch" ("string"), w347) -> (w345:string)
            n123 = call-poly <vilib>:"DAQmx Create Virtual Channel.vi"("task in"=w342, "output terminal configuration"=w344, "physical channels"=w340, "name to assign"=w345, "error in"=w338) -> ("task out"=w341:refnum<k21>, "error out"=w337:errorcluster)  [unwired: 9 in]
          }
          n124 = call-poly <vilib>:"DAQmx Timing.vi"("task/channels in"=w324, "sample mode"=w327, "samples per channel"=100, "rate"=1000.0, "source"=tag "OnboardClock", "error in"=w316) -> ("error out"=w315:errorcluster)  [unwired: 8 in, 1 out]
          n125 = call-poly <vilib>:"DAQmx Write.vi"("task/channels in"=w324, "data"=w319, "error in"=w315) -> ("task out"=w323:refnum<k21>, "error out"=w314:errorcluster)  [unwired: 10 in, 1 out]
          n126 = call <vilib>:"DAQmx Clear Task.vi"("task in"=w323, "error in"=w314) -> ("error out"=w313:errorcluster)  [unwired: 13 in]
        }
      }
    }
    frame "relays" {
      n127 = case shown="\"write\"" w352 {
        tunnel: w356 -> [_ w365]
        tunnel: w355 -> [_ w364]
        tunnel: w351 -> [w357 w362]
        tunnel: [w357 w358] -> w350
        frame "read", Default {
          # "Do nothing, no inputs to read"
        }
        frame "write" {
          # "Allowable device types are AI, AO, Relay, TC, and GPIO (spelling/caps) matters)"
          # "This one works reasonably fast"
          n128 = property class="DAQmx System"() -> ("DevNames"=w371:tag[])  [unwired: 2 in, 2 out]
          n129 = Number To Decimal String(number=w365) -> (decimal integer string=w374:string)  [unwired: 1 in]
          n130 = Concatenate Strings("Relay" ("string"), w374) -> (w373:string)
          n131 = Match First String(2:w371, 3:w373) -> (0:w372:i32)  [unwired: 1 out]
          n132 = Index Array(array=w371, index=w372) -> (element=w370:tag)
          n133 = property class="DAQmx Device"("Active Device"=w370) -> ("DO.Lines"=w367:tag[])  [unwired: 2 in, 2 out]
          n134 = call <vilib>:"DAQmx Create Task.vi"("new task name"="relays task", "error in"=w362) -> ("task out"=w369:refnum<k21>, "error out"=w361:errorcluster)  [unwired: 12 in]
          n135 = for {
            tunnel: w365 -> [w382]
            tunnel: w369 -> [w381]
            tunnel: [w380] -> w363
            tunnel: w367 -> [w379] mode=indexing
            tunnel: w361 -> [w377]
            tunnel: [w376] -> w360
            i -> [w378]
            n136 = Number To Decimal String(number=w382) -> (decimal integer string=w386:string)  [unwired: 1 in]
            n137 = Number To Decimal String(number=w378) -> (decimal integer string=w385:string)  [unwired: 1 in]
            n138 = Concatenate Strings("relayMod" ("string"), w386, "Ch" ("string"), w385) -> (w383:string)
            n139 = call-poly <vilib>:"DAQmx Create Virtual Channel.vi"("task in"=w381, "lines"=w379, "name to assign"=w383, "error in"=w377) -> ("task out"=w380:refnum<k21>, "error out"=w376:errorcluster)  [unwired: 10 in]
          }
          n140 = call-poly <vilib>:"DAQmx Write.vi"("task/channels in"=w363, "data"=w364, "error in"=w360) -> ("task out"=w368:refnum<k21>, "error out"=w359:errorcluster)  [unwired: 10 in, 1 out]
          n141 = call <vilib>:"DAQmx Clear Task.vi"("task in"=w368, "error in"=w359) -> ("error out"=w358:errorcluster)  [unwired: 13 in]
        }
      }
    }
  }
  "Value out" <- w9
  "Bool out" <- w6
  "error out" <- w4
  n142 = call <vilib>:"Simple Error Handler.vi"("error in (no error)"=w4) -> ("error out"=w3:errorcluster)  [unwired: 4 in, 4 out]
  n143 = call <vilib>:"Clear Errors.vi"("error in (no error)"=w3) -> ()  [unwired: 6 in, 1 out]
